vi "图像匹配2.vi"() -> ()   [LabVIEW 2018]
uses:
  <vilib>/vision/NI_Vision_Development_Module.lvlib
panel:
  out "Image 2":T1(plugin-control)
  out "Number of Matches":i32
  out "Matches (pixel)":T2(array[cluster]) {"Bounding Box"."y" format="%.2f"; "Bounding Box"."x" format="%.2f"; "Score" format="%.2f"; "Scale" format="%.2f"; "Angle" format="%.2f"; "Position"."y" format="%.2f"; "Position"."x" format="%.2f"}
  out "error out":errorcluster
  out "Image":T1(plugin-control)
  out "文件名":string[](array[string])
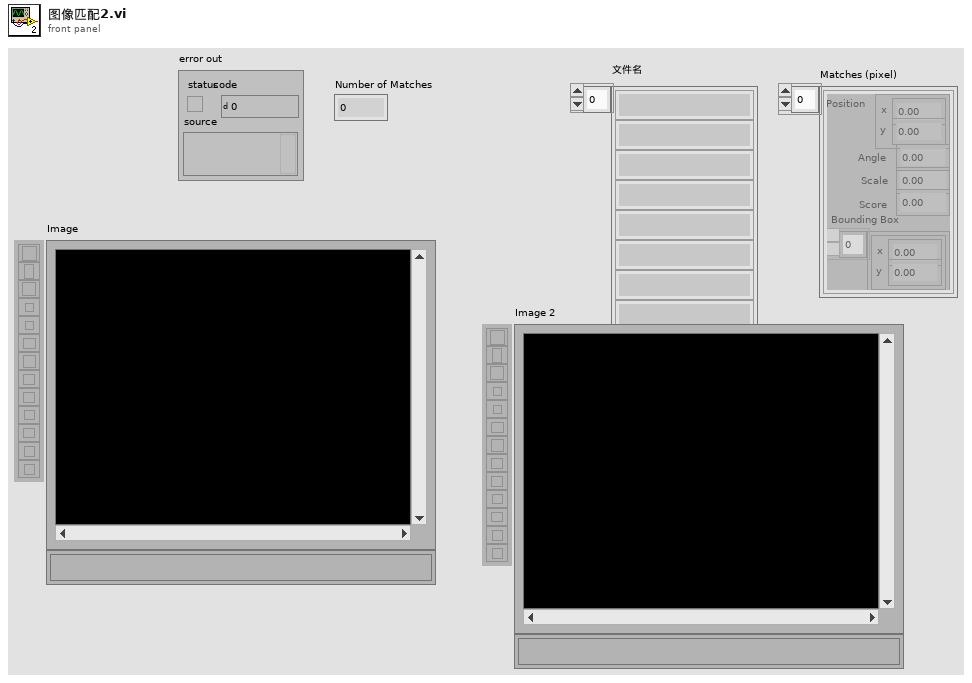
[diagram p1: front panel]
types:
  T1 = typedef "IMAQ Image.ctl" = refnum<image>
  T2 = cluster{"Position":cluster{"x":sgl, "y":sgl}, "Angle":sgl, "Scale":sgl, "Score":sgl, "Bounding Box":cluster{"x":sgl, "y":sgl}[]}[]
  T3 = cluster{"Number of Matches Requested":i32, "Minimum Match Score":sgl, "Angle Ranges":cluster{"Start Angle":sgl, "End Angle":sgl}[]}
  T4 = typedef "Image Type" = u32
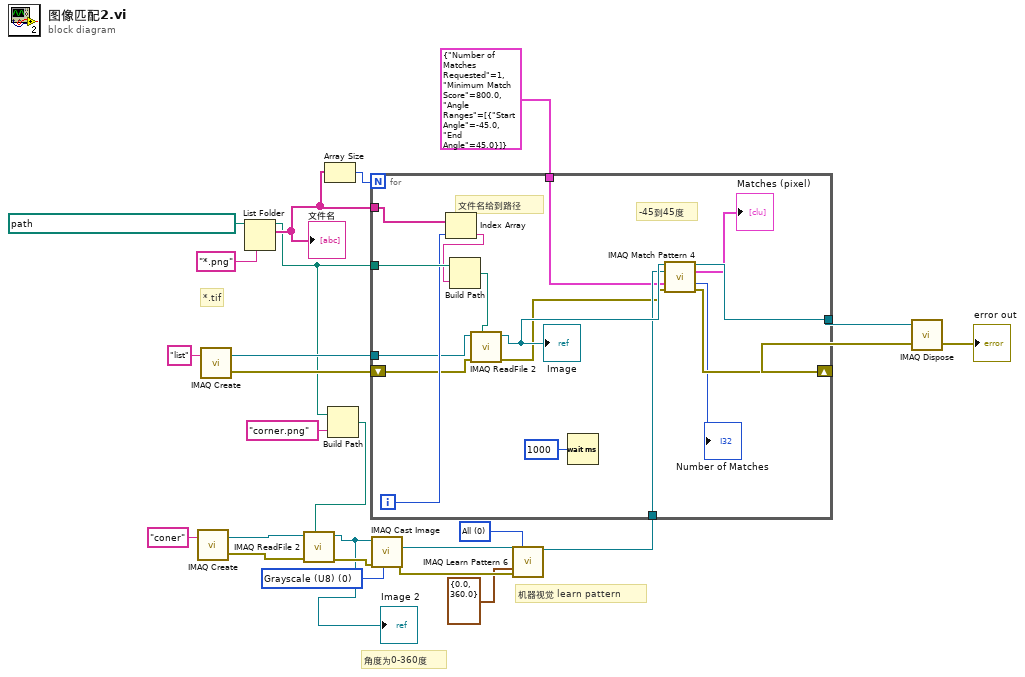
[diagram p0: block diagram]
diagram:
  w5 = 0 items=["All", "Low Discrepancy Sampling", "Grayscale Value Pyramid", "Gradients Pyramid"] ("Algorithm")
  w9 = T4 0 items=["Grayscale (U8)", "Grayscale (I16)", "Grayscale (SGL)", "Complex (CSG)", "RGB (U32)", "HSL (U32)", "RGB (U64)", "Grayscale (U16)"] ("Image Type")
  # "*.tif"
  # "角度为0-360度"
  # "机器视觉 learn pattern"
  n1 = call "IMAQ Create"("Image Name"="coner") -> ("New Image"=w11:T1, "error out"=w10:errorcluster)  [unwired: 4 in]
  n2 = call "IMAQ Create"("Image Name"="list") -> ("New Image"=w23:T1, "error out"=w21:errorcluster)  [unwired: 4 in]
  n3 = List Folder(path=path "D:/Labviewprogram/视觉/Roundcard" ("路径"), pattern="*.png" ("类型")) -> (path out=w15:path, filenames=w17:string[])  [unwired: 2 in, 2 out]
  "文件名" <- w17
  n4 = Array Size(array=w17) -> (size(s)=w16:i32)
  n5 = Build Path(base path=w15, name or relative path="corner.png" ("名称或相对路径")) -> (appended path=w12:path)
  n6 = call "IMAQ ReadFile 2"("File Path"=w12, "error in (no error)"=w10, "Image"=w11) -> ("error out"=w8:errorcluster, "Image Out"=w2:T1)  [unwired: 4 in, 3 out]
  "Image 2" <- w2
  n7 = call "IMAQ Cast Image"("Image Type"=w9, "error in (no error)"=w8, "Image Src"=w2) -> ("error out"=w6:errorcluster, "Image Dst Out"=w7:T1)  [unwired: 7 in]
  n8 = call "IMAQ Learn Pattern 6"("Image"=w7, "Algorithm"=w5, "Angle Range"=cluster{"Start Angle":sgl, "End Angle":sgl} {"Start Angle"=0.0, "End Angle"=360.0}, "error in (no error)"=w6) -> ("Template Image Out"=w3:T1)  [unwired: 9 in, 2 out]
  n9 = for {
    N: w16 -> [_]
    tunnel: w17 -> [w41]
    tunnel: w15 -> [w40]
    tunnel: w23 -> [w37]
    shift-right: [w31] -> w19
    shift-left: w21 -> [w36]
    tunnel: [w30] -> w20
    tunnel: w3 -> [w33]
    tunnel: T3 {"Number of Matches Requested"=1, "Minimum Match Score"=800.0, "Angle Ranges"=[{"Start Angle"=-45.0, "End Angle"=45.0}]} -> [w26]
    i -> [w39]
    # "-45到45度"
    # "文件名给到路径"
    n10 = Index Array(array=w41, index=w39) -> (element=w38:string)
    n11 = Build Path(base path=w40, name or relative path=w38) -> (appended path=w27:path)
    n12 = call "IMAQ ReadFile 2"("File Path"=w27, "error in (no error)"=w36, "Image"=w37) -> ("error out"=w32:errorcluster, "Image Out"=w34:T1)  [unwired: 4 in, 3 out]
    "Image" <- w34
    n13 = Wait (ms)(milliseconds to wait=u32 1000 ("等待时间（毫秒）")) -> ()  [unwired: 1 out]
    n14 = call "IMAQ Match Pattern 4"("Image"=w34, "Template Image"=w33, "Parameters"=w26, "error in (no error)"=w32) -> ("Image (duplicate)"=w30:T1, "Matches (pixel)"=→"Matches (pixel)":T2, "Number of Matches"=→"Number of Matches":i32, "error out"=w31:errorcluster)  [unwired: 7 in, 1 out]
  }
  n15 = call "IMAQ Dispose"("Image"=w20, "error in (no error)"=w19) -> ("error out"=→"error out":errorcluster)  [unwired: 4 in]
